vi "spilib_setbitsperword.vi"(8 "error in (no error)":errorcluster, 10 "bits per word":u8, 11 "handle":i32) -> (0 "error out":errorcluster, 3 "handle out":i32)   [LabVIEW 2017]
uses:
  <vilib>/Utility/error.llb/Error Cluster From Error Code.vi
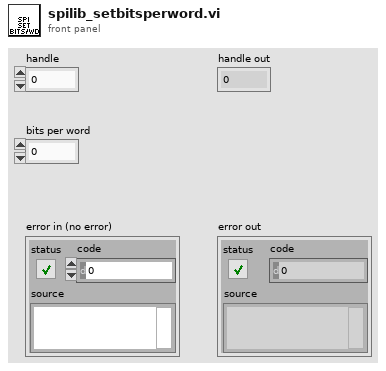
[diagram p1: front panel]
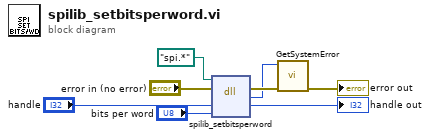
[diagram p0: block diagram]
diagram:
  n1 = dll-call lib="?" fn="spilib_setbitsperword"(path in=path "spi.*", error in="error in (no error)", "handle"="handle", "bpw"="bits per word") -> (error out=w7:errorcluster, "return type"=w5:i32, "handle"=→"handle out":i32)  [unwired: 2 in, 1 out]
  n2 = call <vilib>:"GetSystemError.vi"("error in (no error)"=w7, "Retval"=w5) -> ("error out"=→"error out":errorcluster)  [unwired: 9 in]
